vi "VL53L0X_InitializeI2C.vi"(10 "Port":T1, 11 "REV2mDistanceSensorDevRef":T2) -> (3 "REV2mDistanceSensorDevRef Out":T2)   [LabVIEW 2019, in "DistanceSensorDriver.lvlib"]
uses:
  DistanceSensorDriver.lvlib
  Typedef/REV2mDistanceSensorDevRef.ctl
  Typedef/Ports.ctl
panel:
  out "Init I2C Status":i32
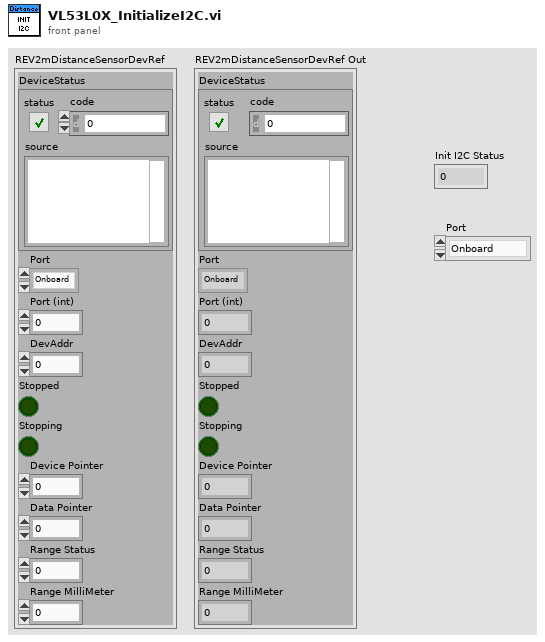
[diagram p1: front panel]
types:
  T1 = typedef "DistanceSensorDriver.lvlib/Ports.ctl" = enum32{"Onboard", "MXP"}
  T2 = typedef "DistanceSensorDriver.lvlib/REV2mDistanceSensorDevRef.ctl" = cluster{"DeviceStatus":errorcluster, "Port":T1, "Port (int)":i32, "DevAddr":i32, "Stopped":bool, "Stopping":bool, "Device Pointer":u64, "Data Pointer":u64, "Range Status":u8, "Range MilliMeter":u16}
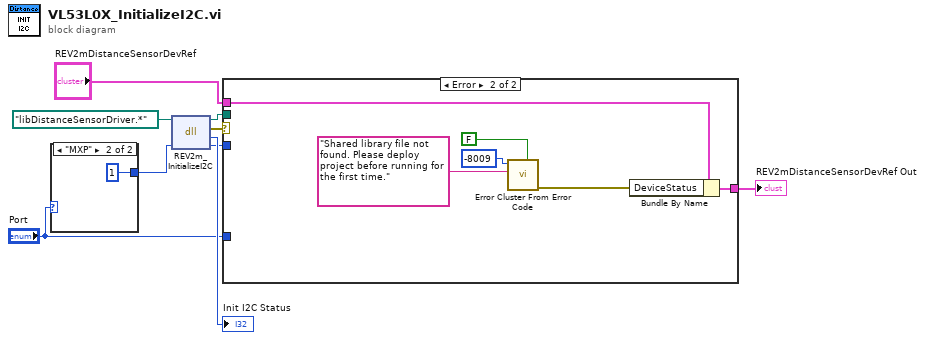
[diagram p0: block diagram]
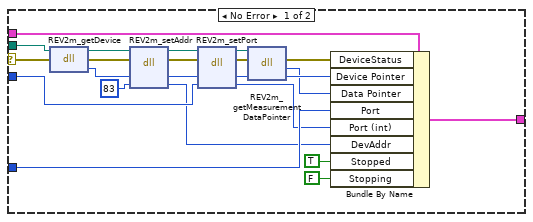
[diagram p2: hidden frame]
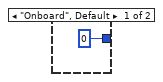
[diagram p3: hidden frame]
diagram:
  n1 = case shown="\"MXP\"" "Port" {
    tunnel: [0 ("port") 1 ("port")] -> w7
    frame "Onboard", Default {
    }
    frame "MXP" {
    }
  }
  n2 = dll-call lib="?" fn="REV2m_InitializeI2C"(path in=path "libDistanceSensorDriver.*", "port"=w7) -> (path out=w2:path, error out=w1:errorcluster, "Status"=→"Init I2C Status":i32, "port"=w6:i32)  [unwired: 2 in]
  n3 = case shown="Error" w1 {
    selector: w1 -> [w12 _]
    tunnel: w6 -> [w34 _]
    tunnel: "Port" -> [w33 _]
    tunnel: [w32 w35] -> w4
    tunnel: "REV2mDistanceSensorDevRef" -> [w31 w37]
    tunnel: w2 -> [w14 _]
    frame No Error {
      n4 = dll-call lib="?" fn="REV2m_getDevice"(path in=w14, error in=w12) -> (path out=w29:path, error out=w28:errorcluster, "Dev"=w30:u64)  [unwired: 1 in]
      n5 = dll-call lib="?" fn="REV2m_setAddr"(path in=w29, error in=w28, "Dev"=w30, "addr"=83) -> (path out=w26:path, error out=w25:errorcluster, "Dev"=w23:u64, "addr"=w22:i32)  [unwired: 2 in]
      n6 = dll-call lib="?" fn="REV2m_setPort"(path in=w26, error in=w25, "Dev"=w23, "port"=w34) -> (path out=w19:path, error out=w18:errorcluster, "Dev"=w17:u64, "port"=w24:i32)  [unwired: 2 in]
      n7 = dll-call lib="?" fn="REV2m_getMeasurementDataPointer"(path in=w19, error in=w18, "Dev"=w17) -> (error out=w13:errorcluster, "return type"=w15:u64, "Dev"=w16:u64)  [unwired: 1 in, 1 out]
      n8 = Bundle By Name(cluster=w31, "DeviceStatus"=w13, "Device Pointer"=w16, "Data Pointer"=w15, "Port"=w33, "Port (int)"=w24, "DevAddr"=w22, "Stopped"=TRUE, "Stopping"=FALSE) -> (w32:T2)
    }
    frame Error {
      n9 = call <vilib>:"Error Cluster From Error Code.vi"("is warning? (False)"=FALSE, "error message (\"\")"="Shared library file not found. Please deploy project before running for the first time." ("format string"), "error code (0)"=-8009) -> ("error out"=w36:errorcluster)  [unwired: 6 in]
      n10 = Bundle By Name(cluster=w37, "DeviceStatus"=w36) -> (w35:T2)
    }
  }
  "REV2mDistanceSensorDevRef Out" <- w4
